vi "Main.vi"() -> ()   [LabVIEW 2016, in "SimpleCalculator.lvlib"]
doc: "This calculator contains the basic operations like Addition, Subraction, Multiplication and Division. It also contains Square operaton."
uses:
  SimpleCalculator.lvlib
panel:
  in  "Square Root":bool caption="Multiply"
  in  "Square":bool caption="Multiply"
  in  "Stop":bool
  in  "Divide":bool
  in  "Multiply":bool
  in  "Subtract":bool
  in  "Add":bool
  out "Output":dbl
  in  "Input 2":dbl
  in  "Input 1":dbl
  # "Simple Calculator"
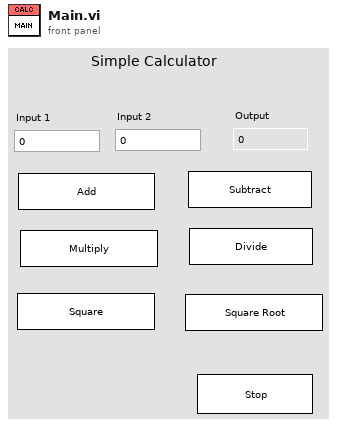
[diagram p1: front panel]
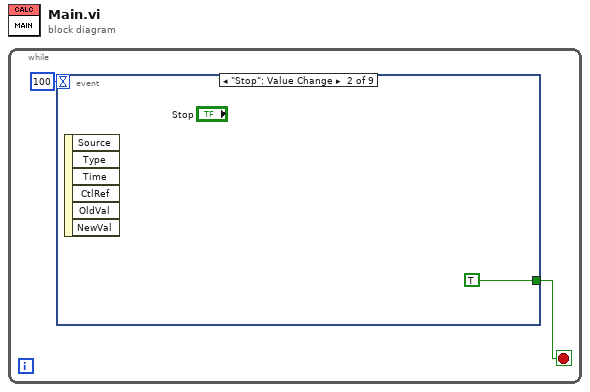
[diagram p0: block diagram]
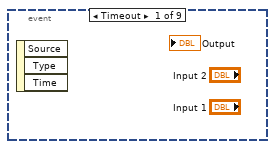
[diagram p2: hidden frame]
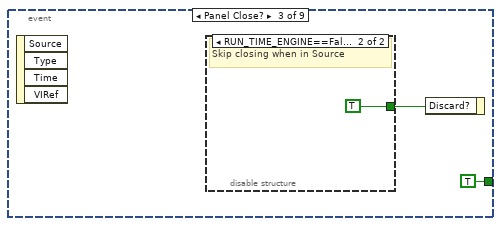
[diagram p3: hidden frame]
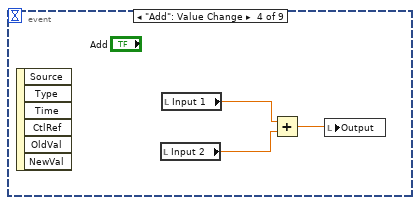
[diagram p5: hidden frame]
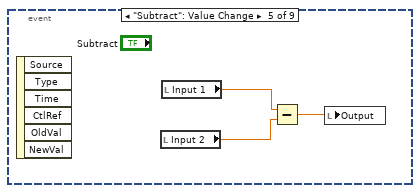
[diagram p6: hidden frame]
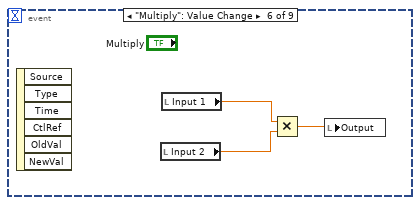
[diagram p7: hidden frame]
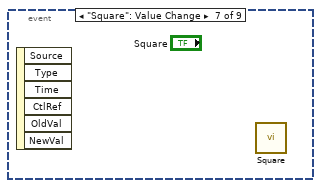
[diagram p8: hidden frame]
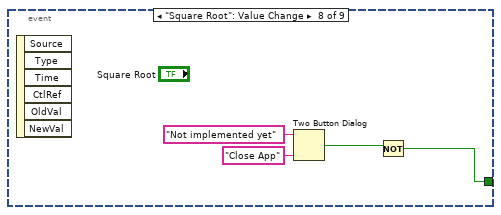
[diagram p9: hidden frame]
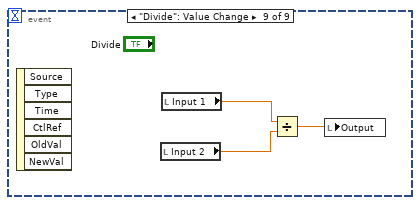
[diagram p10: hidden frame]
diagram:
  n1 = while {
    stop <- w1 stop-if-true
    n2 = event shown="[1] \"Stop\": Value Change" {
      selector: _ -> [_ _ _ _ _ _ _ _ _]
      dyn-events: _ -> [_ _ _ _ _ _ _ _ _]
      timeout: 100 -> [_ _ _ _ _ _ _ _ _]
      tunnel: [_ TRUE TRUE _ _ _ _ w16 _] -> w1
      event Timeout {
        n3 = event-data() -> ()  [unwired: 1 in, 3 out]
      }
      event "Stop": Value Change {
        n4 = event-data() -> ()  [unwired: 1 in, 6 out]
      }
      event Panel Close? {
        n5 = event-data() -> ()  [unwired: 1 in, 4 out]
        n6 = disable-structure shown="RUN_TIME_ENGINE==False" {
          disable-tunnel: [_ TRUE] -> w4
          frame condition #0 {
          }
          frame condition #1 (active) {
            # "Skip closing when in Source"
          }
        }
        n7 = event-data("Discard?"=w4) -> ()  [unwired: 1 in, 1 out]
      }
      event "Add": Value Change {
        n8 = event-data() -> ()  [unwired: 1 in, 6 out]
        n9 = local read "Input 2"() -> (w8:dbl)
        n10 = local read "Input 1"() -> (w9:dbl)
        n11 = Add(x=w9, y=w8) -> (x+y=w7:dbl)
        n12 = local write "Output"(w7) -> ()
      }
      event "Subtract": Value Change {
        n13 = event-data() -> ()  [unwired: 1 in, 6 out]
        n14 = local read "Input 2"() -> (w11:dbl)
        n15 = local read "Input 1"() -> (w12:dbl)
        n16 = Subtract(x=w12, y=w11) -> (x-y=w10:dbl)
        n17 = local write "Output"(w10) -> ()
      }
      event "Multiply": Value Change {
        n18 = event-data() -> ()  [unwired: 1 in, 6 out]
        n19 = local read "Input 2"() -> (w14:dbl)
        n20 = local read "Input 1"() -> (w15:dbl)
        n21 = Multiply(x=w15, y=w14) -> (x*y=w13:dbl)
        n22 = local write "Output"(w13) -> ()
      }
      event "Square": Value Change {
        n23 = event-data() -> ()  [unwired: 1 in, 6 out]
        n24 = call "Square.vi"() -> ()  [unwired: 12 in]
      }
      event "Square Root": Value Change {
        n25 = event-data() -> ()  [unwired: 1 in, 6 out]
        n26 = Two Button Dialog(message="Not implemented yet", 1:"Close App" ("F button name (\"Cancel\")")) -> (T button?=w17:bool)  [unwired: 1 in]
        n27 = Not(x=w17) -> (.not. x?=w16:bool)
      }
      event "Divide": Value Change {
        n28 = event-data() -> ()  [unwired: 1 in, 6 out]
        n29 = local read "Input 2"() -> (w21:dbl)
        n30 = local read "Input 1"() -> (w22:dbl)
        n31 = Divide(x=w22, y=w21) -> (x/y=w20:dbl)
        n32 = local write "Output"(w20) -> ()
      }
    }
  }
